vi "Read Total A-scans per volume.vi"(8 "error in (no error)":errorcluster, 11 "Scan in":refnum<class "Scan.lvclass">) -> (0 "error out":errorcluster, 2 "Total A-scans per volume":dbl=900.0, 3 "Scan out":refnum<class "Scan.lvclass">)   [LabVIEW 2017, in "Scan.lvclass"]
uses:
  Scan.lvclass
  Scan.lvclass/Scan.ctl
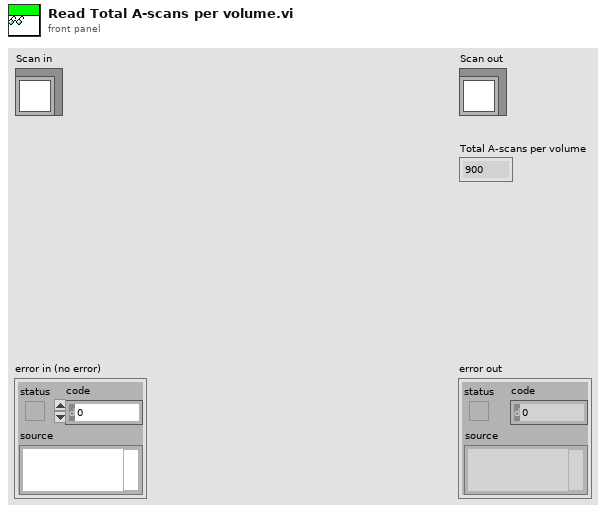
[diagram p1: front panel]
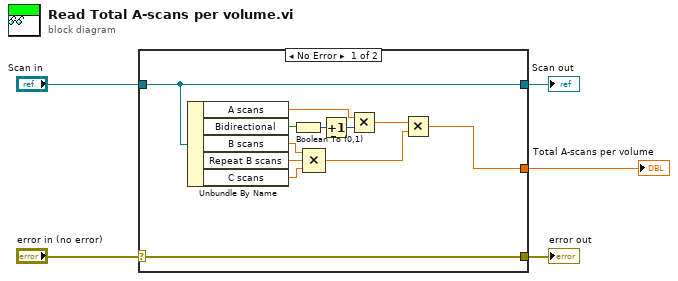
[diagram p0: block diagram]
diagram:
  n1 = case shown="No Error" "error in (no error)" {
    selector: "error in (no error)" -> [w17 w18]
    tunnel: [w17 w18] -> w4
    tunnel: [w16 w19] -> w2
    tunnel: "Scan in" -> [w16 w19]
    tunnel: [w6 _] -> w1
    frame No Error {
      n2 = Unbundle By Name(w16) -> ("A scans"=w12:dbl, "Bidirectional"=w13:bool, "B scans"=w11:dbl, "Repeat B scans"=w10:dbl, "C scans"=w9:dbl)
      n3 = Boolean To (0,1)(Boolean=w13) -> (0, 1=w15:i16)
      n4 = Compound Arithmetic op=MULTIPLY(w11, w10, w9) -> (w7:dbl)
      n5 = Increment(x=w15) -> (x+1=w14:i16)
      n6 = Multiply(x=w12, y=w14) -> (x*y=w8:dbl)
      n7 = Multiply(x=w8, y=w7) -> (x*y=w6:dbl)
    }
    frame Error {
    }
  }
  "error out" <- w4
  "Scan out" <- w2
  "Total A-scans per volume" <- w1
